vi "Send Message.vi"(5 "return data? (F)":bool, 7 "action":T1, 8 "error in (no error)":errorcluster, 11 "send data":variant) -> (0 "error out":errorcluster, 3 "return data":variant)   [LabVIEW 2018, in "GLog.lvlib" / "Registry.lvlib"]
uses:
  Registry.lvlib
  Registry Actions.ctl
  Registry Message.ctl
  Registry Actions Event.vi
  <vilib>/Utility/error.llb/Error Cluster From Error Code.vi
  <vilib>/ErrorRing/Error Ring.xnode
  reuse_library/Utilities/Utilities.lvlib
panel:
  # "Connector Pane"
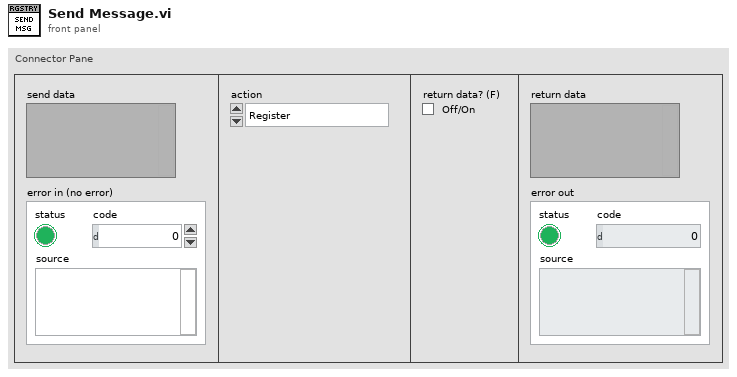
[diagram p1: front panel]
types:
  T1 = typedef "GLog.lvlib/Registry.lvlib/Registry Actions.ctl" = enum16{"Register", "Log", "Enable", "Enable All", "Disable", "Disable All", "List", "Unregister", "Unregister All", "Shutdown"}
  T2 = typedef "GLog.lvlib/Registry.lvlib/Registry Message.ctl" = cluster{"action":T1, "data":variant, "return notifier":refnum<notifier>}
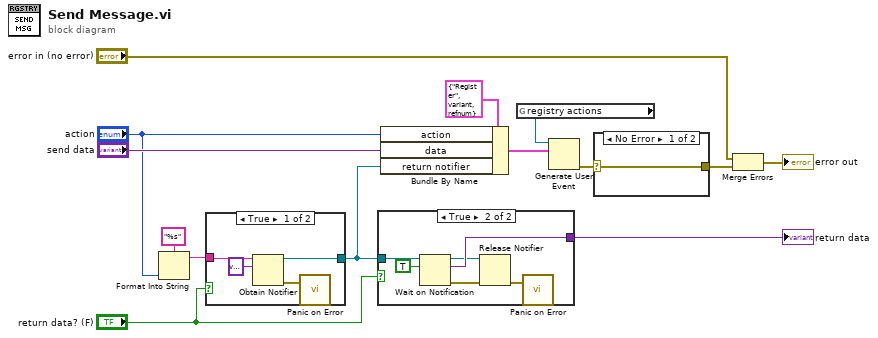
[diagram p0: block diagram]
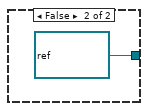
[diagram p2: hidden frame]
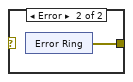
[diagram p3: hidden frame]
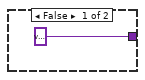
[diagram p4: hidden frame]
diagram:
  n1 = Format Into String(format string="%s", "action") -> (resulting string=w6:string)  [unwired: 2 in, 1 out]
  n2 = case shown="True" "return data? (F)" {
    tunnel: [w17 refnum<notifier> refnum ("notifier out")] -> w7
    tunnel: w6 -> [w16 _]
    frame True {
      n3 = Obtain Notifier(name (unnamed)=w16, notification data type=variant ("element data type")) -> (notifier out=w17:refnum<notifier>, error out=w18:errorcluster)  [unwired: 2 in, 1 out]
      n4 = call "Panic on Error.vi"("error in (no error)"=w18) -> ()  [unwired: 3 in]
    }
    frame False {
    }
  }
  n5 = case shown="True" "return data? (F)" {
    tunnel: w7 -> [_ w26]
    tunnel: [variant w25] -> w13
    frame False {
    }
    frame True {
      n6 = Wait on Notification(notifier=w26, ignore previous (F)=TRUE) -> (notifier out=w24:refnum<notifier>, notification=w25:variant, error out=w23:errorcluster)  [unwired: 2 in, 1 out]
      n7 = Release Notifier(notifier=w24, error in (no error)=w23) -> (error out=w22:errorcluster)  [unwired: 1 in, 2 out]
      n8 = call "Panic on Error.vi"("error in (no error)"=w22) -> ()  [unwired: 3 in]
    }
  }
  "return data" <- w13
  n9 = Bundle By Name(cluster=T2 {"action"=enum."Register", "data"=variant, "return notifier"=refnum} ("registry message"), "action"="action", "data"="send data", "return notifier"=w7) -> (w9:T2)
  n10 = global read "Registry Actions Event.vi" "registry actions"() -> (w4:refnum<user-event>)
  n11 = Generate User Event(user event=w4, event data cluster=w9) -> (error out=w3:errorcluster)  [unwired: 2 in, 1 out]
  n12 = case shown="No Error" w3 {
    selector: w3 -> [w27 _]
    tunnel: [w27 w28] -> w10
    frame No Error {
    }
    frame Error {
      n13 = xnode "Error Ring"() -> ("error out"=w28:errorcluster)
    }
  }
  n14 = Merge Errors("error in (no error)", w10) -> (→"error out":errorcluster)
